vi "fgv_range_tables.vi"(4 "Range Checking":bool=TRUE, 5 "Attribute Value in (0.0)":dbl, 6 "Range Tables (Empty)":T1(array[cluster]) {"Type" items=["Range", "Coerced", "Discrete"]}, 7 "Operation":T2(ring)=enum."Check", 8 "error in":errorcluster, 10 "Range Table ID in":string, 11 "Query String in (\"\")":string) -> (0 "error out":errorcluster, 1 "Numeric I32 Value out":i32, 2 "Default value out":string, 3 "Enum output":string)   [LabVIEW 2014, in "rszvl_rsidr_core.lvlib"]
uses:
  rszvl_rsidr_core.lvlib
  type_Error_Codes.ctl
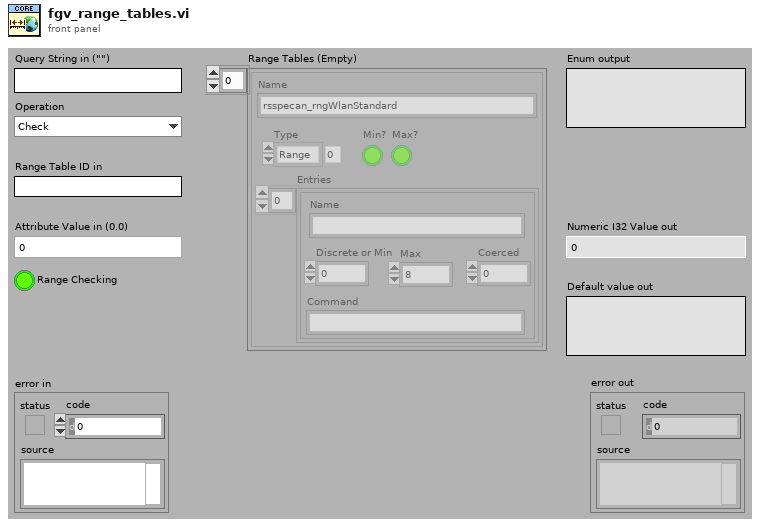
[diagram p1: front panel]
types:
  T1 = cluster{"Name":string, "Type":i32, "Min?":bool, "Max?":bool, "Entries":cluster{"Name":string, "Discrete or Min":dbl, "Max":dbl, "Coerced":dbl, "Command":string}[]}[]
  T2 = enum16{"Initialize", "Check", "Get Numeric Value", "Get Default Value"}
  T3 = typedef "rszvl_rsidr_core.lvlib/type_Error_Codes.ctl" = enum16{"No_error", "VISA_err_ResourceNotFound", "VISA_err_Timeout", "VISA_warn_MoreDataAvailable", "RS_err_MissingCallback", "RS_err_InvalidAttribute", "RS_err_InvalidValue", "RS_err_UnknownResource", "RS_err_AlreadyInitialized", "RS_err_InstrumentStatus", "RS_err_BadRepCapName", "RS_err_TypesMismatch", "RS_err_ValueNotSupported", "RS_err_InvalidRngTable", "RS_err_IDqueryFail", "RS_err_UnexpResponse", "VISA_warn_ConfigNotLoaded", "RS_err_AttributeNotReadable", "RS_err_AttributeNotWritable", "RS_err_InstrumentType", "RS_err_InstrumentOption", "VISA_err_InvalidSize", "RS_err_ReliabilityIndicator", "VISA_warn_UnknownStatus", "VISA_warn_TermCharRead", "VISA_err_IO_error"}
  T4 = cluster{"Name":string, "Discrete or Min":dbl, "Max":dbl, "Coerced":dbl, "Command":string}[]
  T5 = cluster{"Name":string, "Discrete or Min":dbl, "Max":dbl, "Coerced":dbl, "Command":string}
  T6 = cluster{"Name":string, "Type":i32, "Variant":variant}
  T7 = cluster{"Name":string, "Type":i32, "Variant":variant}[]
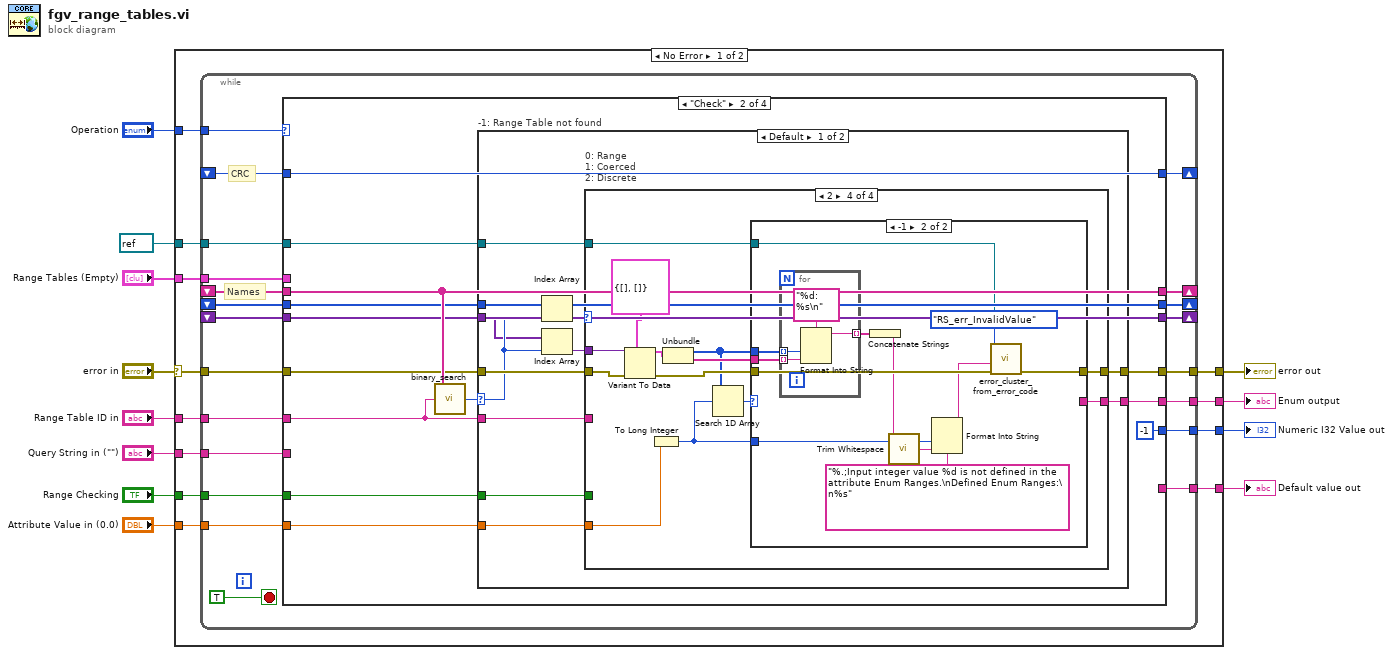
[diagram p0: block diagram]
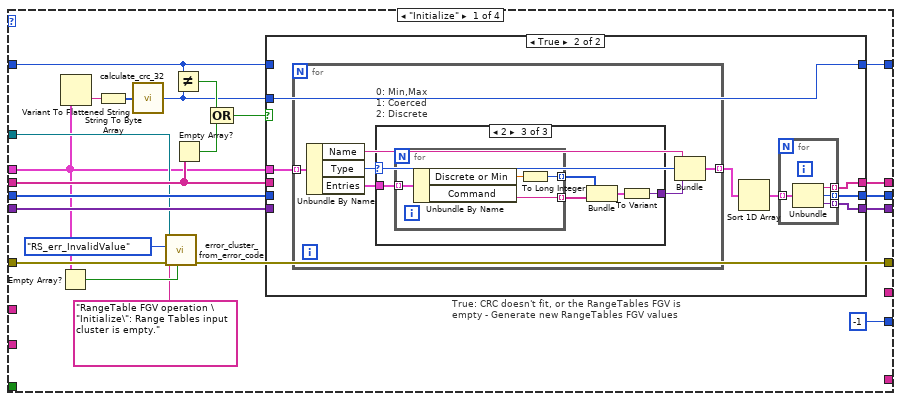
[diagram p2: hidden frame]
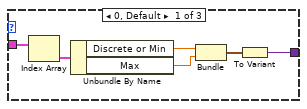
[diagram p4: hidden frame]
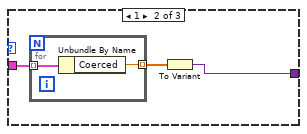
[diagram p5: hidden frame]
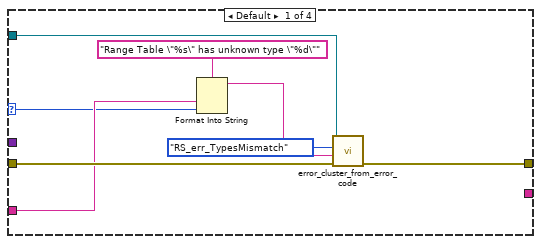
[diagram p6: hidden frame]
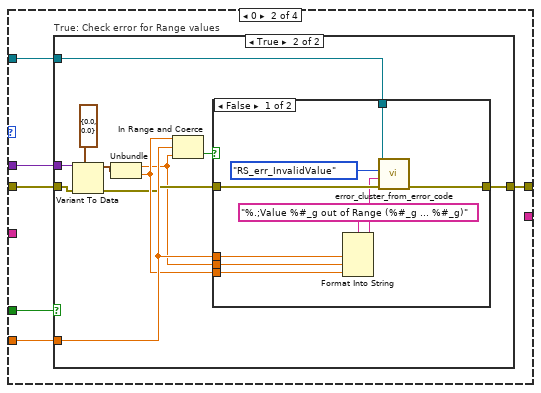
[diagram p7: hidden frame]
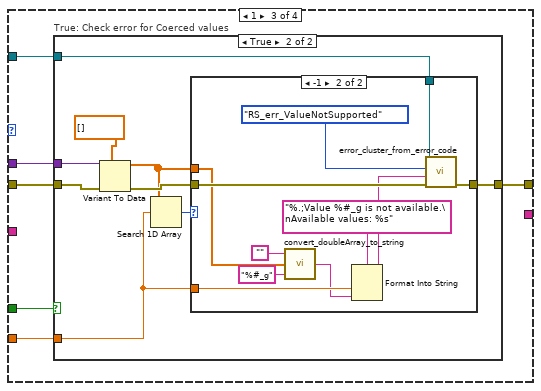
[diagram p10: hidden frame]
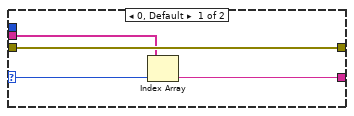
[diagram p13: hidden frame]
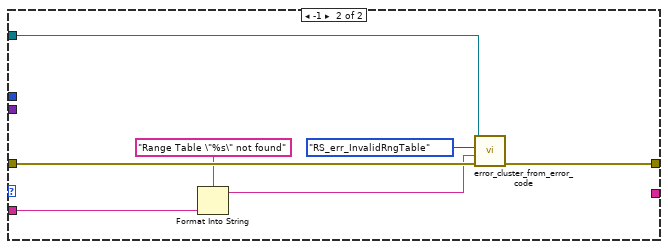
[diagram p14: hidden frame]
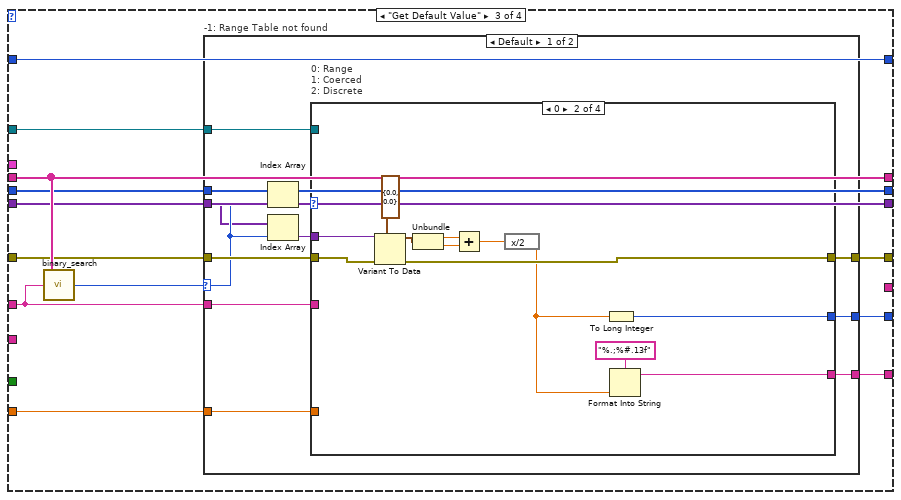
[diagram p15: hidden frame]
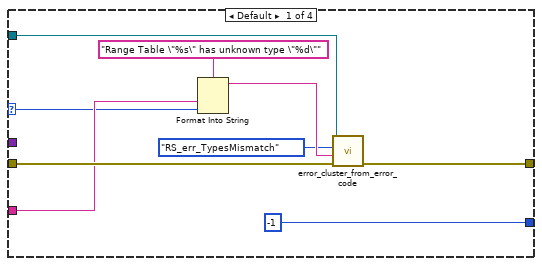
[diagram p16: hidden frame]
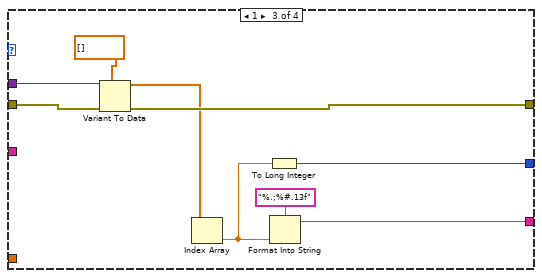
[diagram p17: hidden frame]
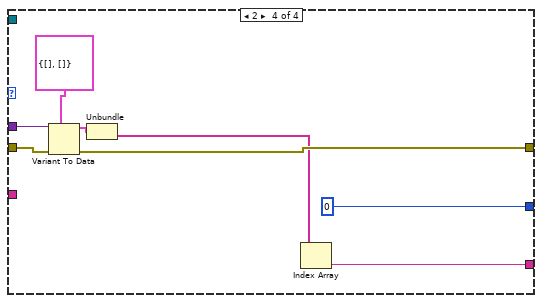
[diagram p18: hidden frame]
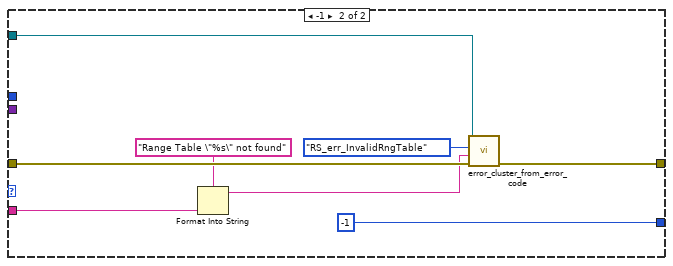
[diagram p19: hidden frame]
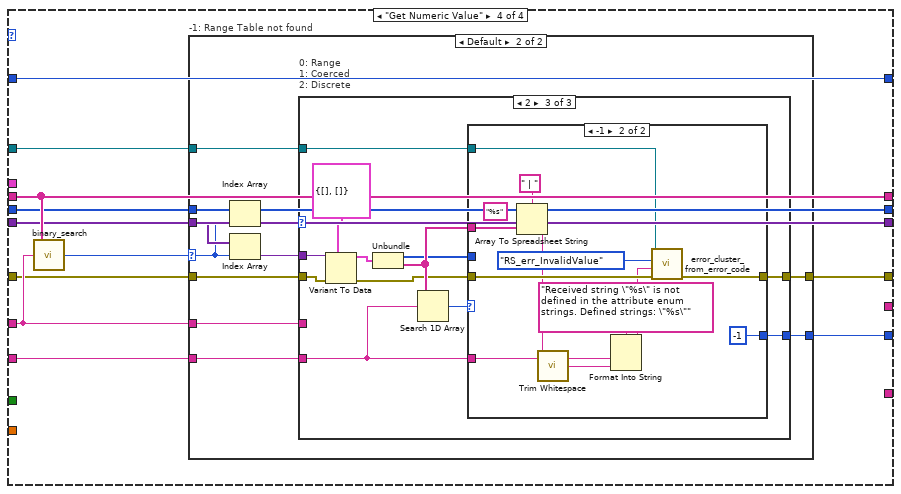
[diagram p20: hidden frame]
diagram:
  n1 = case shown="No Error" "error in" {
    selector: "error in" -> [w18 w376]
    tunnel: "Operation" -> [w24 _]
    tunnel: [w17 w376] -> w5
    tunnel: "Range Table ID in" -> [w23 _]
    tunnel: "Attribute Value in (0.0)" -> [w22 _]
    tunnel: "Query String in (\"\")" -> [w21 _]
    tunnel: [w20 -1] -> w7
    tunnel: "Range Checking" -> [w19 _]
    tunnel: [w16 _] -> w4
    tunnel: [w15 _] -> w3
    tunnel: refnum<visa-resource-name> refnum ("VISA resource name") -> [w14 _]
    tunnel: "Range Tables (Empty)" -> [w13 _]
    frame No Error {
      n2 = while {
        tunnel: w24 -> [w45]
        tunnel: w23 -> [w44]
        tunnel: w22 -> [w43]
        tunnel: w21 -> [w42]
        tunnel: [w41] -> w20
        tunnel: w19 -> [w40]
        tunnel: w18 -> [w39]
        tunnel: [w38] -> w17
        tunnel: [w37] -> w16
        shift-right: [w35] -> _
        shift-left: _ -> [w36]
        shift-right: [w32] -> _
        shift-left: _ -> [w33]
        shift-right: [w31] -> _
        shift-left: _ -> [w30]
        tunnel: [w29] -> w15
        shift-right: [w27] -> _
        shift-left: _ -> [w28]
        tunnel: w14 -> [w26]
        tunnel: w13 -> [w25]
        stop <- TRUE stop-if-true
        # "CRC"
        # "Names"
        n3 = case shown="\"Check\"" w45 {
          tunnel: [w64 w121 w249 w318] -> w38
          tunnel: w44 -> [_ w109 w247 w314]
          tunnel: w42 -> [_ _ _ w316]
          tunnel: [-1 -1 w238 w317] -> w41
          tunnel: w40 -> [_ w118 _ _]
          tunnel: w43 -> [_ w119 w248 _]
          tunnel: w39 -> [w63 w115 w245 w313]
          tunnel: [_ w117 _ _] -> w37
          tunnel: w36 -> [w58 w112 w242 w311]
          tunnel: [w66 w112 w242 w311] -> w35
          tunnel: w33 -> [w57 w114 w244 w310]
          tunnel: [w65 w114 w244 w310] -> w32
          tunnel: [w62 w116 w246 w315] -> w31
          tunnel: w30 -> [w55 w116 w246 w315]
          tunnel: [_ _ w241 _] -> w29
          tunnel: w28 -> [w52 w111 w240 w309]
          tunnel: [w51 w111 w240 w309] -> w27
          tunnel: w26 -> [w47 w110 w239 w308]
          tunnel: w25 -> [w46 _ _ _]
          frame "Initialize" {
            n4 = Empty Array?(array=w46) -> (empty?=w56:bool)
            n5 = Variant To Flattened String(Variant=w46) -> (data string=w61:string)  [unwired: 1 out]
            n6 = String To Byte Array(string=w61) -> (unsigned byte array=w60:u8[])
            n7 = call "calculate_crc_32.vi"("Data in"=w60) -> ("CRC_32"=w50:u32)  [unwired: 4 in]
            n8 = call "error_cluster_from_error_code.vi"("error creation enabled (T)"=w56, "error in"=w63, "error message (\"\")"="RangeTable FGV operation \"Initialize\": Range Tables input cluster is empty." ("format string"), "Error Enum in"=type_Error_Codes."RS_err_InvalidValue", "VISA resource name"=w47) -> ("error out"=w64:errorcluster)  [unwired: 5 in, 1 out]
            n9 = Not Equal?(x=w52, y=w50) -> (x != y?=w54:bool)
            n10 = Empty Array?(array=w55) -> (empty?=w53:bool)
            n11 = Compound Arithmetic op=OR(w54, w53) -> (w59:bool)
            n12 = case "True: CRC doesn't fit, or the RangeTables FGV is empty - Generate new RangeTables FGV values" shown="True" w59 {
              tunnel: [w70 w77] -> w66
              tunnel: [w69 w76] -> w65
              tunnel: w46 -> [_ w74]
              tunnel: [w71 w73] -> w62
              tunnel: w55 -> [w71 _]
              tunnel: w58 -> [w70 _]
              tunnel: w57 -> [w69 _]
              tunnel: w52 -> [w68 _]
              tunnel: [w68 w72] -> w51
              tunnel: w50 -> [_ w72]
              frame False {
              }
              frame True {
                n13 = for {
                  tunnel: w74 -> [w88] mode=indexing
                  tunnel: [w83] -> w78 mode=indexing
                  n14 = Unbundle By Name(w88) -> ("Name"=w86:string, "Type"=w85:i32, "Entries"=w87:T4)
                  n15 = case "0: Min,Max\n1: Coerced\n2: Discrete" shown="2" w85 {
                    tunnel: w87 -> [w94 w97 w104]
                    tunnel: [w89 w95 w103] -> w84
                    frame 0, Default {
                      n16 = Index Array(array=w94) -> (element=w93:T5)  [unwired: 1 in]
                      n17 = Unbundle By Name(w93) -> ("Discrete or Min"=w91:dbl, "Max"=w92:dbl)
                      n18 = Bundle("Discrete or Min"=w91, "Max"=w92) -> (w90:cluster{"Discrete or Min":dbl, "Max":dbl})  [unwired: 1 in]
                      n19 = To Variant(anything=w90) -> (Variant=w89:variant)
                    }
                    frame 1 {
                      n20 = for {
                        tunnel: [w99] -> w96 mode=indexing
                        tunnel: w97 -> [w98] mode=indexing
                        n21 = Unbundle By Name(w98) -> ("Coerced"=w99:dbl)
                      }
                      n22 = To Variant(anything=w96) -> (Variant=w95:variant)
                    }
                    frame 2 {
                      n23 = for {
                        tunnel: w104 -> [w108] mode=indexing
                        tunnel: [w107] -> w101 mode=indexing
                        tunnel: [w105] -> w100 mode=indexing
                        n24 = Unbundle By Name(w108) -> ("Discrete or Min"=w106:dbl, "Command"=w107:string)
                        n25 = To Long Integer(number=w106) -> (32bit integer=w105:i32)
                      }
                      n26 = Bundle(w100, w101) -> (w102:cluster{i32[], string[]})  [unwired: 1 in]
                      n27 = To Variant(anything=w102) -> (Variant=w103:variant)
                    }
                  }
                  n28 = Bundle("Name"=w86, "Type"=w85, "Variant"=w84) -> (w83:T6)  [unwired: 1 in]
                }
                n29 = Sort 1D Array(array=w78) -> (sorted array=w75:T7)
                n30 = for {
                  tunnel: w75 -> [w81] mode=indexing
                  tunnel: [w82] -> w73 mode=indexing
                  tunnel: [w80] -> w77 mode=indexing
                  tunnel: [w79] -> w76 mode=indexing
                  n31 = Unbundle(w81) -> ("Name"=w82:string, "Type"=w80:i32, "Variant"=w79:variant)
                }
              }
            }
          }
          frame "Check" {
            n32 = call "binary_search.vi"("String to search"=w109, "Strings in"=w116) -> ("Index out"=w113:i32)  [unwired: 3 in]
            n33 = case "-1: Range Table not found" shown="Default" w113 {
              selector: w113 -> [w127 _]
              tunnel: [w132 w237] -> w121
              tunnel: w115 -> [w131 w236]
              tunnel: w119 -> [w133 _]
              tunnel: w118 -> [w130 _]
              tunnel: [w124 _] -> w117
              tunnel: w109 -> [w123 w235]
              tunnel: w114 -> [w126 _]
              tunnel: w112 -> [w129 _]
              tunnel: w110 -> [w122 w231]
              frame Default {
                n34 = Index Array(array=w129, index=w127) -> (element=w128:i32)
                n35 = Index Array(array=w126, index=w127) -> (element=w125:variant)
                n36 = case "0: Range\n1: Coerced\n2: Discrete" shown="2" w128 {
                  selector: w128 -> [w137 _ _ _]
                  tunnel: w133 -> [_ w146 w175 w200]
                  tunnel: [w139 w147 w173 w205] -> w132
                  tunnel: w131 -> [w140 w144 w172 w210]
                  tunnel: w130 -> [_ w145 w174 _]
                  tunnel: w125 -> [_ w143 w171 w209]
                  tunnel: [_ _ _ w201] -> w124
                  tunnel: w123 -> [w138 _ _ _]
                  tunnel: w122 -> [w134 w142 w170 w198]
                  frame Default {
                    n37 = Format Into String(format string="Range Table \"%s\" has unknown type \"%d\"" ("string"), w138, w137) -> (resulting string=w136:string)  [unwired: 2 in, 1 out]
                    n38 = call "error_cluster_from_error_code.vi"("error in"=w140, "error message (\"\")"=w136, "Error Enum in"=type_Error_Codes."RS_err_TypesMismatch", "VISA resource name"=w134) -> ("error out"=w139:errorcluster)  [unwired: 6 in, 1 out]
                  }
                  frame 0 {
                    n39 = case "True: Check error for Range values" shown="True" w145 {
                      tunnel: w146 -> [_ w158]
                      tunnel: [w148 w157] -> w147
                      tunnel: w144 -> [w148 w152]
                      tunnel: w143 -> [_ w153]
                      tunnel: w142 -> [_ w149]
                      frame False {
                      }
                      frame True {
                        n40 = Variant To Data(error in=w152, type=cluster{"Min":dbl, "Max":dbl} {"Min"=0.0, "Max"=0.0} ("output cluster"), Variant=w153) -> (data=w154:cluster{"Min":dbl, "Max":dbl}, error out=w151:errorcluster)
                        n41 = Unbundle(w154) -> ("Min"=w150:dbl, "Max"=w156:dbl)
                        n42 = In Range and Coerce(upper limit=w156, x=w158, lower limit=w150) -> (In Range?=w159:bool)  [unwired: 1 out]
                        n43 = case shown="False" w159 {
                          tunnel: w158 -> [w167 _]
                          tunnel: w151 -> [w166 w169]
                          tunnel: [w165 w169] -> w157
                          tunnel: w150 -> [w164 _]
                          tunnel: w156 -> [w163 _]
                          tunnel: w149 -> [w160 _]
                          frame False {
                            n44 = Format Into String(format string="%.;Value %#_g out of Range (%#_g ... %#_g)" ("string"), w167, w164, w163) -> (resulting string=w162:string)  [unwired: 2 in, 1 out]
                            n45 = call "error_cluster_from_error_code.vi"("error in"=w166, "error message (\"\")"=w162, "Error Enum in"=type_Error_Codes."RS_err_InvalidValue", "VISA resource name"=w160) -> ("error out"=w165:errorcluster)  [unwired: 6 in, 1 out]
                          }
                          frame True {
                          }
                        }
                      }
                    }
                  }
                  frame 1 {
                    n46 = case "True: Check error for Coerced values" shown="True" w174 {
                      tunnel: w175 -> [_ w185]
                      tunnel: w172 -> [w176 w181]
                      tunnel: [w176 w183] -> w173
                      tunnel: w171 -> [_ w180]
                      tunnel: w170 -> [_ w178]
                      frame False {
                      }
                      frame True {
                        n47 = Variant To Data(error in=w181, type=dbl[] [], Variant=w180) -> (data=w177:dbl[], error out=w179:errorcluster)
                        n48 = Search 1D Array(1D array=w177, element=w185) -> (index of element=w184:i32)  [unwired: 1 in]
                        n49 = case shown="-1" w184 {
                          tunnel: w185 -> [_ w196]
                          tunnel: w179 -> [w186 w195]
                          tunnel: [w186 w194] -> w183
                          tunnel: w178 -> [_ w192]
                          tunnel: w177 -> [_ w190]
                          frame 0, Default {
                          }
                          frame -1 {
                            n50 = call "convert_doubleArray_to_string.vi"("Format string (%.;%#.12g)"="%#_g", "double array in"=w190, "String to add before (\"\")"="" ("Empty String Constant")) -> ("string out"=w189:string)  [unwired: 2 in]
                            n51 = Format Into String(format string="%.;Value %#_g is not available.\nAvailable values: %s" ("string"), w196, w189) -> (resulting string=w193:string)  [unwired: 2 in, 1 out]
                            n52 = call "error_cluster_from_error_code.vi"("error in"=w195, "error message (\"\")"=w193, "Error Enum in"=type_Error_Codes."RS_err_ValueNotSupported", "VISA resource name"=w192) -> ("error out"=w194:errorcluster)  [unwired: 6 in, 1 out]
                          }
                        }
                      }
                    }
                  }
                  frame 2 {
                    n53 = Variant To Data(error in=w210, type=cluster{i32[], string[]} {[], []} ("anything"), Variant=w209) -> (data=w207:cluster{i32[], string[]}, error out=w206:errorcluster)
                    n54 = To Long Integer(number=w200) -> (32bit integer=w203:i32)
                    n55 = Unbundle(w207) -> (w199:i32[], w202:string[])
                    n56 = Search 1D Array(1D array=w199, element=w203) -> (index of element=w204:i32)  [unwired: 1 in]
                    n57 = case shown="-1" w204 {
                      selector: w204 -> [w213 _]
                      tunnel: w203 -> [_ w225]
                      tunnel: w206 -> [w214 w224]
                      tunnel: [w214 w223] -> w205
                      tunnel: w202 -> [w212 w221]
                      tunnel: [w211 _] -> w201
                      tunnel: w199 -> [_ w222]
                      tunnel: w198 -> [_ w215]
                      frame 0, Default {
                        n58 = Index Array(array=w212, index=w213) -> (element=w211:string)
                      }
                      frame -1 {
                        n59 = for {
                          tunnel: w222 -> [w230] mode=indexing
                          tunnel: w221 -> [w229] mode=indexing
                          tunnel: [w227] -> w220 mode=indexing
                          n60 = Format Into String(format string="%d: %s\n", w230, w229) -> (resulting string=w227:string)  [unwired: 2 in, 1 out]
                        }
                        n61 = Concatenate Strings(w220) -> (w219:string)
                        n62 = call "Trim Whitespace.vi"("string"=w219) -> ("trimmed string"=w218:string)  [unwired: 1 in]
                        n63 = Format Into String(format string="%.;Input integer value %d is not defined in the attribute Enum Ranges.\nDefined Enum Ranges:\n%s" ("string"), w225, w218) -> (resulting string=w217:string)  [unwired: 2 in, 1 out]
                        n64 = call "error_cluster_from_error_code.vi"("error in"=w224, "error message (\"\")"=w217, "Error Enum in"=type_Error_Codes."RS_err_InvalidValue", "VISA resource name"=w215) -> ("error out"=w223:errorcluster)  [unwired: 6 in, 1 out]
                      }
                    }
                  }
                }
              }
              frame -1 {
                n65 = Format Into String(format string="Range Table \"%s\" not found" ("string"), w235) -> (resulting string=w233:string)  [unwired: 2 in, 1 out]
                n66 = call "error_cluster_from_error_code.vi"("error in"=w236, "error message (\"\")"=w233, "Error Enum in"=type_Error_Codes."RS_err_InvalidRngTable", "VISA resource name"=w231) -> ("error out"=w237:errorcluster)  [unwired: 6 in, 1 out]
              }
            }
          }
          frame "Get Default Value" {
            n67 = call "binary_search.vi"("String to search"=w247, "Strings in"=w246) -> ("Index out"=w243:i32)  [unwired: 3 in]
            n68 = case "-1: Range Table not found" shown="Default" w243 {
              selector: w243 -> [w256 _]
              tunnel: [w260 w307] -> w249
              tunnel: w245 -> [w259 w306]
              tunnel: w248 -> [w261 _]
              tunnel: w247 -> [w253 w305]
              tunnel: w244 -> [w255 _]
              tunnel: w242 -> [w258 _]
              tunnel: [w252 _] -> w241
              tunnel: w239 -> [w251 w301]
              tunnel: [w250 -1] -> w238
              frame Default {
                n69 = Index Array(array=w258, index=w256) -> (element=w257:i32)
                n70 = Index Array(array=w255, index=w256) -> (element=w254:variant)
                n71 = case "0: Range\n1: Coerced\n2: Discrete" shown="0" w257 {
                  selector: w257 -> [w266 _ _ _]
                  tunnel: w261 -> [_ _ _ _]
                  tunnel: [w268 w275 w288 w294] -> w260
                  tunnel: w259 -> [w269 w282 w291 w299]
                  tunnel: w254 -> [_ w281 w290 w298]
                  tunnel: w253 -> [w267 _ _ _]
                  tunnel: [_ w273 w285 w295] -> w252
                  tunnel: w251 -> [w263 _ _ _]
                  tunnel: [-1 w271 w283 0] -> w250
                  frame Default {
                    n72 = Format Into String(format string="Range Table \"%s\" has unknown type \"%d\"" ("string"), w267, w266) -> (resulting string=w265:string)  [unwired: 2 in, 1 out]
                    n73 = call "error_cluster_from_error_code.vi"("error in"=w269, "error message (\"\")"=w265, "Error Enum in"=type_Error_Codes."RS_err_TypesMismatch", "VISA resource name"=w263) -> ("error out"=w268:errorcluster)  [unwired: 6 in, 1 out]
                  }
                  frame 0 {
                    n74 = Variant To Data(error in=w282, type=cluster{"Min":dbl, "Max":dbl} {"Min"=0.0, "Max"=0.0} ("output cluster"), Variant=w281) -> (data=w279:cluster{"Min":dbl, "Max":dbl}, error out=w275:errorcluster)
                    n75 = Unbundle(w279) -> ("Min"=w278:dbl, "Max"=w277:dbl)
                    n76 = Add(x=w278, y=w277) -> (x+y=w276:dbl)
                    n77 = expression code="x/2"(w276) -> (w272:dbl)
                    n78 = To Long Integer(number=w272) -> (32bit integer=w271:i32)
                    n79 = Format Into String(format string="%.;%#.13f", w272) -> (resulting string=w273:string)  [unwired: 2 in, 1 out]
                  }
                  frame 1 {
                    n80 = Variant To Data(error in=w291, type=dbl[] [], Variant=w290) -> (data=w287:dbl[], error out=w288:errorcluster)
                    n81 = Index Array(array=w287) -> (element=w284:dbl)  [unwired: 1 in]
                    n82 = To Long Integer(number=w284) -> (32bit integer=w283:i32)
                    n83 = Format Into String(format string="%.;%#.13f", w284) -> (resulting string=w285:string)  [unwired: 2 in, 1 out]
                  }
                  frame 2 {
                    n84 = Variant To Data(error in=w299, type=cluster{i32[], string[]} {[], []} ("anything"), Variant=w298) -> (data=w296:cluster{i32[], string[]}, error out=w294:errorcluster)
                    n85 = Unbundle(w296) -> (w293:string[])  [unwired: 1 out]
                    n86 = Index Array(array=w293) -> (element=w295:string)  [unwired: 1 in]
                  }
                }
              }
              frame -1 {
                n87 = Format Into String(format string="Range Table \"%s\" not found" ("string"), w305) -> (resulting string=w303:string)  [unwired: 2 in, 1 out]
                n88 = call "error_cluster_from_error_code.vi"("error in"=w306, "error message (\"\")"=w303, "Error Enum in"=type_Error_Codes."RS_err_InvalidRngTable", "VISA resource name"=w301) -> ("error out"=w307:errorcluster)  [unwired: 6 in, 1 out]
              }
            }
          }
          frame "Get Numeric Value" {
            n89 = call "binary_search.vi"("String to search"=w314, "Strings in"=w315) -> ("Index out"=w312:i32)  [unwired: 3 in]
            n90 = case "-1: Range Table not found" shown="Default" w312 {
              selector: w312 -> [_ w328]
              tunnel: [w323 w336] -> w318
              tunnel: [_ w335] -> w317
              tunnel: w316 -> [_ w334]
              tunnel: w314 -> [w322 w333]
              tunnel: w313 -> [w324 w332]
              tunnel: w311 -> [_ w331]
              tunnel: w310 -> [_ w329]
              tunnel: w308 -> [w319 w326]
              frame -1 {
                n91 = Format Into String(format string="Range Table \"%s\" not found" ("string"), w322) -> (resulting string=w321:string)  [unwired: 2 in, 1 out]
                n92 = call "error_cluster_from_error_code.vi"("error in"=w324, "error message (\"\")"=w321, "Error Enum in"=type_Error_Codes."RS_err_InvalidRngTable", "VISA resource name"=w319) -> ("error out"=w323:errorcluster)  [unwired: 6 in, 1 out]
              }
              frame Default {
                n93 = Index Array(array=w331, index=w328) -> (element=w330:i32)
                n94 = Index Array(array=w329, index=w328) -> (element=w327:variant)
                n95 = case "0: Range\n1: Coerced\n2: Discrete" shown="2" w330 {
                  selector: w330 -> [w342 _ _]
                  tunnel: [w343 w345 w358] -> w336
                  tunnel: [_ w346 w359] -> w335
                  tunnel: w334 -> [_ w347 w356]
                  tunnel: w332 -> [w344 w345 w354]
                  tunnel: w333 -> [w341 _ _]
                  tunnel: w327 -> [_ _ w353]
                  tunnel: w326 -> [w337 _ w348]
                  frame Default {
                    n96 = Format Into String(format string="Range Table \"%s\" has unknown type \"%d\"" ("string"), w341, w342) -> (resulting string=w338:string)  [unwired: 2 in, 1 out]
                    n97 = call "error_cluster_from_error_code.vi"("error in"=w344, "error message (\"\")"=w338, "Error Enum in"=type_Error_Codes."RS_err_TypesMismatch", "VISA resource name"=w337) -> ("error out"=w343:errorcluster)  [unwired: 6 in, 1 out]
                  }
                  frame 0, 1 {
                    n98 = call "convert_string_to_int32.vi"("String in"=w347) -> ("int32 value out"=w346:i32)  [unwired: 4 in]
                  }
                  frame 2 {
                    n99 = Variant To Data(error in=w354, type=cluster{i32[], string[]} {[], []} ("anything"), Variant=w353) -> (data=w355:cluster{i32[], string[]}, error out=w349:errorcluster)
                    n100 = Unbundle(w355) -> (w350:i32[], w351:string[])
                    n101 = Search 1D Array(1D array=w351, element=w356) -> (index of element=w357:i32)  [unwired: 1 in]
                    n102 = case shown="-1" w357 {
                      selector: w357 -> [w362 _]
                      tunnel: [_ w375] -> w358
                      tunnel: [w360 -1] -> w359
                      tunnel: w349 -> [_ w373]
                      tunnel: w356 -> [_ w374]
                      tunnel: w351 -> [_ w371]
                      tunnel: w350 -> [w361 _]
                      tunnel: w348 -> [_ w363]
                      frame 0, Default {
                        n103 = Index Array(array=w361, index=w362) -> (element=w360:i32)
                      }
                      frame -1 {
                        n104 = Array To Spreadsheet String(delimiter (Tab)=" | ", array=w371, 3:"%s" ("format string")) -> (spreadsheet string=w367:string)
                        n105 = call "Trim Whitespace.vi"("string"=w367) -> ("trimmed string"=w366:string)  [unwired: 1 in]
                        n106 = Format Into String(format string="Received string \"%s\" is not defined in the attribute enum strings. Defined strings: \"%s\"", w374, w366) -> (resulting string=w365:string)  [unwired: 2 in, 1 out]
                        n107 = call "error_cluster_from_error_code.vi"("error in"=w373, "error message (\"\")"=w365, "Error Enum in"=type_Error_Codes."RS_err_InvalidValue", "VISA resource name"=w363) -> ("error out"=w375:errorcluster)  [unwired: 6 in, 1 out]
                      }
                    }
                  }
                }
              }
            }
          }
        }
      }
    }
    frame Error {
    }
  }
  "error out" <- w5
  "Enum output" <- w4
  "Numeric I32 Value out" <- w7
  "Default value out" <- w3
